vi "Reply Msg DataSocket.vi"(8 "error in (no error)":errorcluster, 11 "Target Reply Time Test Actor in":refnum<class "Target Reply Time Test Actor.lvclass">) -> (0 "error out":errorcluster, 2 "Variant":variant, 3 "Target Reply Time Test Actor out":refnum<class "Target Reply Time Test Actor.lvclass">)   [LabVIEW 2023, in "Target Reply Time Test Actor.lvlib" / "Target Reply Time Test Actor.lvclass"]
uses:
  Target Reply Time Test Actor.lvclass
  Target Reply Time Test Actor.lvclass/Target Reply Time Test Actor.ctl
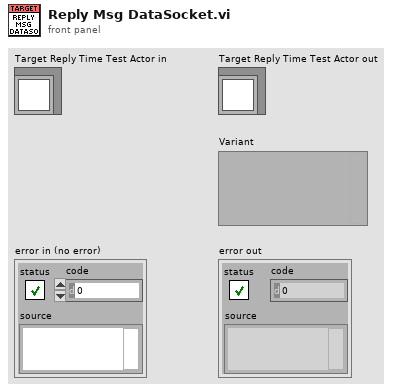
[diagram p1: front panel]
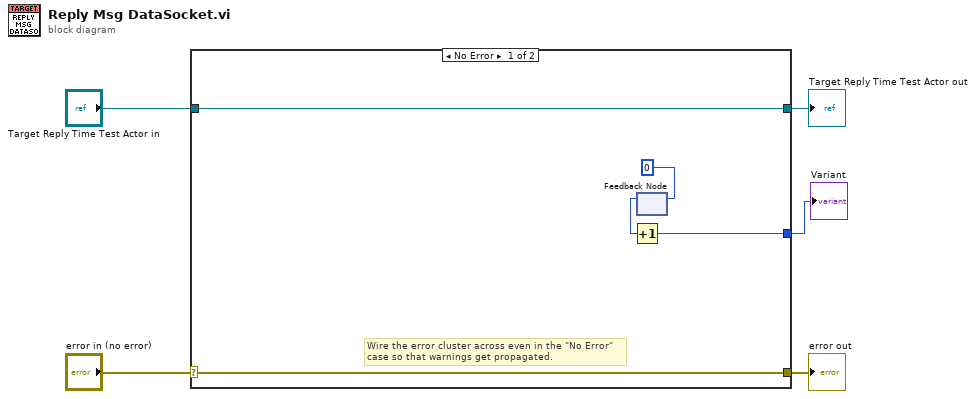
[diagram p0: block diagram]
diagram:
  n1 = case shown="No Error" "error in (no error)" {
    selector: "error in (no error)" -> [w9 w12]
    tunnel: [w9 w12] -> w4
    tunnel: [w10 w11] -> w2
    tunnel: "Target Reply Time Test Actor in" -> [w10 w11]
    tunnel: [w6 _] -> w1
    frame No Error {
      # "Wire the error cluster across even in the \"No Error\"\ncase so that warnings get propagated."
      n2 = feedback-in #1(0) -> ()
      n3 = feedback #1() -> (w7:i32)  [unwired: 1 in]
      n4 = Increment(x=w7) -> (x+1=w6:i32)
    }
    frame Error {
    }
  }
  "error out" <- w4
  "Target Reply Time Test Actor out" <- w2
  "Variant" <- w1
